vi "Initialize.vi"(7 "error in (no error)":errorcluster caption="错误输入（无错误）", 10 "PanelLinkNode 输入":refnum<class "PanelLinkNode.lvclass"> caption="LinkNode in") -> (0 "error out":errorcluster caption="错误输出", 2 "SelfNode*":refnum<data-value>)   [LabVIEW 2013, in "PanelLinkNode.lvclass"]
uses:
  PanelLinkNode.lvclass
  PanelLinkNode.lvclass/PanelLinkNode.ctl
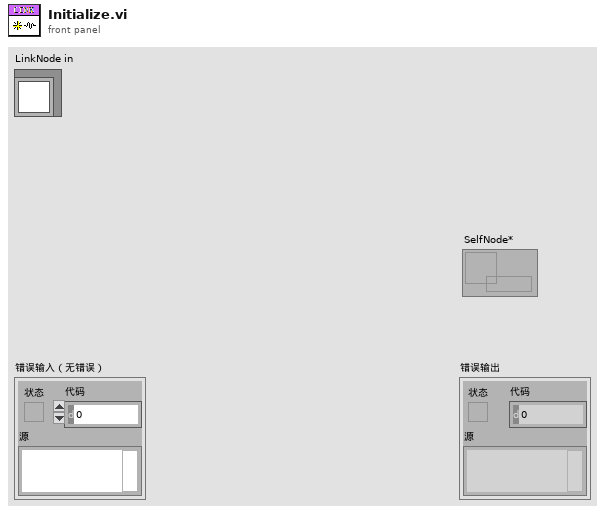
[diagram p1: front panel]
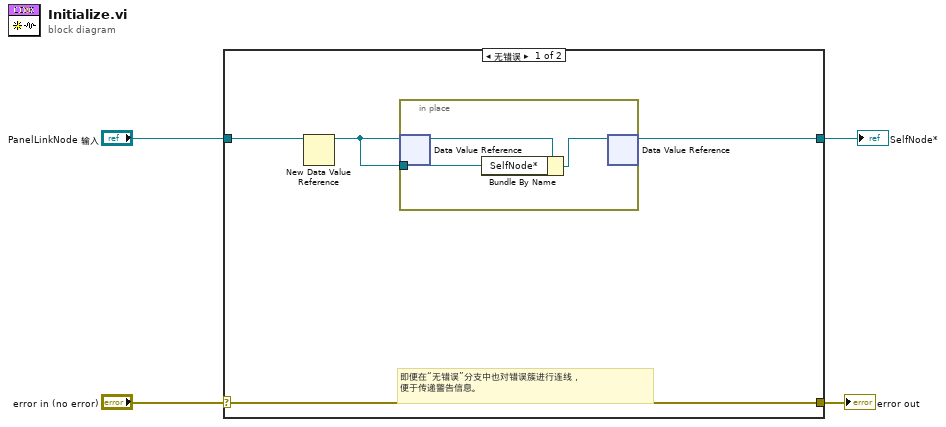
[diagram p0: block diagram]
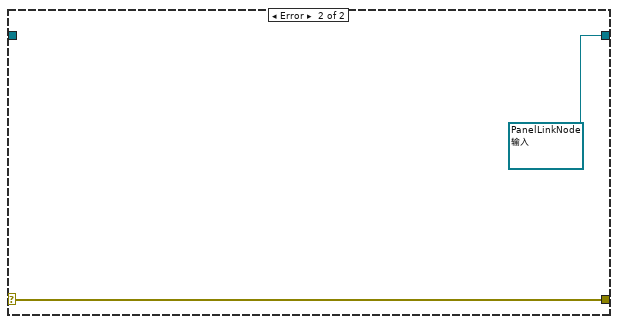
[diagram p2: hidden frame]
diagram:
  n1 = case shown="无错误" "error in (no error)" {
    selector: "error in (no error)" -> [w8 w13]
    tunnel: [w8 w13] -> w3
    tunnel: "PanelLinkNode 输入" -> [w7 _]
    tunnel: [w5 refnum<data-value> refnum ("data value reference")] -> w1
    frame No Error {
      # "即便在“无错误”分支中也对错误簇进行连线，\n便于传递警告信息。"
      n2 = New Data Value Reference(data value=w7) -> (data value reference=w6:refnum<data-value>)  [unwired: 1 in, 1 out]
      n3 = in-place {
        in-place-border: w6 -> [w10]
        n4 = in-place-dvr #1(w6) -> (w11:refnum<class "PanelLinkNode.lvclass">)  [unwired: 1 out]
        n5 = Bundle By Name(cluster=w11, "SelfNode*"=w10) -> (w9:refnum<class "PanelLinkNode.lvclass">)
        n6 = in-place-dvr #1(w9) -> (w5:refnum<data-value>)  [unwired: 1 out]
      }
    }
    frame Error {
    }
  }
  "error out" <- w3
  "SelfNode*" <- w1
